vi "BatteryShift.vi"(1 "Battery Level":dbl format="%#_13g", 2 "Gear":enum16{"HIGH", "LOW"}(ring)) -> (0 "Gear":enum16{"HIGH", "LOW"}(ring))   [LabVIEW 2017]
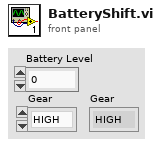
[diagram p1: front panel]
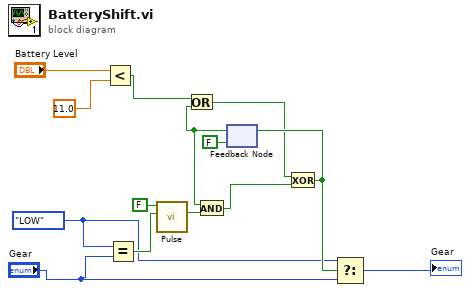
[diagram p0: block diagram]
diagram:
  w6 = enum16{"HIGH", "LOW"}."LOW" ("Enum 3")
  n1 = Less?(x="Battery Level", y=11.0) -> (x < y?=w12:bool)
  n2 = Equal?(x=w6, y="Gear") -> (x = y?=w8:bool)
  n3 = call "Pulse.vi"("Input"=w8, "Rising Edge?"=FALSE) -> ("Output"=w4:bool)  [unwired: 9 in]
  n4 = feedback #1(FALSE) -> (w3:bool)
  n5 = Or(x=w12, y=w3) -> (x .or. y?=w10:bool)
  n6 = And(x=w3, y=w4) -> (x .and. y?=w2:bool)
  n7 = Exclusive Or(1:w2, 2:w10) -> (0:w11:bool)
  n8 = feedback-in #1(w11) -> ()
  n9 = Select(t=w6, s=w11, f="Gear") -> (s? t:f=→"Gear":enum16{"HIGH", "LOW"})
